vi "Auto Cross.vi"(9 "Defense":T1(ring), 10 "arm":refnum<class "arm.lvclass">, 11 "drive":refnum<class "drive.lvclass">) -> (1 "Stop Wheels":bool, 2 "arm":refnum<class "arm.lvclass">, 3 "drive":refnum<class "drive.lvclass">)   [LabVIEW 2015]
uses:
  drive/drive.lvclass
  arm/arm.lvclass
  <vilib>/Rock Robotics/WPI/RobotDrive/WPI_RobotDriveArcadeDrive_Standard(NoSaturation).vi
  Robot Global Data.vi
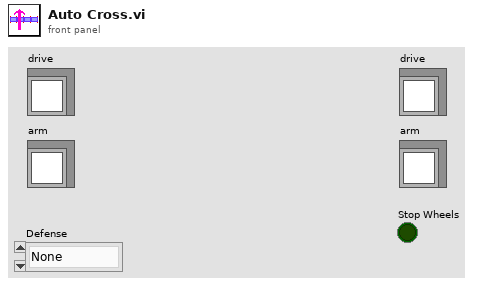
[diagram p1: front panel]
types:
  T1 = enum16{"None", "Low Bar", "Porticullis", "CDF", "Ramparts", "Moat", "Drawbridge", "Sally Port", "Rock Wall", "Rough Terrain"}
  T2 = typedef "WPI_PotentiometerDevRef.ctl" = cluster{"DevStatus":errorcluster, "Analog Channel":T3, "Invert Output":bool}
  T3 = typedef "FPGA_AIChannel.ctl" = enum8{"AI 0", "AI 1", "AI 2", "AI 3", "AI MXP 0", "AI MXP 1", "AI MXP 2", "AI MXP 3", "Invalid"}
  T4 = typedef "WPI_RobotDriveDevRef.ctl" = cluster{"DevStatus":errorcluster, "Motors[]":T5[], "Square Inputs":bool, "Max Output":dbl}
  T5 = typedef "WPI_MotorControlDeviceRef.ctl" = cluster{"DeviceStatus":errorcluster, "Type":T6, "PWM":cluster{"PWM Channel":T7, "DeadBand":T8}, "CAN":cluster{"Device Number":u8, "Control Mode":T9, "Semaphore":T10, "Max Vout":dbl, "TalonSRX Control Mode":T11}, "Invert":bool}
  T6 = typedef "WPI_MotorControlType.ctl" = enum16{"PWM", "CAN", "CANTalonSRX"}
  T7 = typedef "FPGA_DIOPWMChannel.ctl" = enum8{"PWM 0", "PWM 1", "PWM 2", "PWM 3", "PWM 4", "PWM 5", "PWM 6", "PWM 7", "PWM 8", "PWM 9", "PWM MXP 0", "PWM MXP 1", "PWM MXP 2", "PWM MXP 3", "PWM MXP 4", "PWM MXP 5", "PWM MXP 6", "PWM MXP 7", "PWM MXP 8", "PWM MXP 9", "Invalid"}
  T8 = typedef "WPI_PWMDeadband.ctl" = cluster{"Name":string, "maxPositivePwm":i32, "minPositivePwm":i32, "centerPwm":i32, "maxNegativePwm":i32, "minNegativePwm":i32, "angularRange":u16}
  T9 = typedef "WPI_CANJaguar_ControlMode.ctl" = enum8{"Percent VBus", "Current", "Speed", "Position", "Voltage"}
  T10 = typedef "Semaphore RefNum" = refnum<k1>
  T11 = typedef "WPI_CANTalonSRX_APIControlMode.ctl" = enum8{"Percent VBus", "Speed", "Position", "Slave", "Unchanged / Invalid", "Voltage Compensation", "Current", "Motion Profile"}
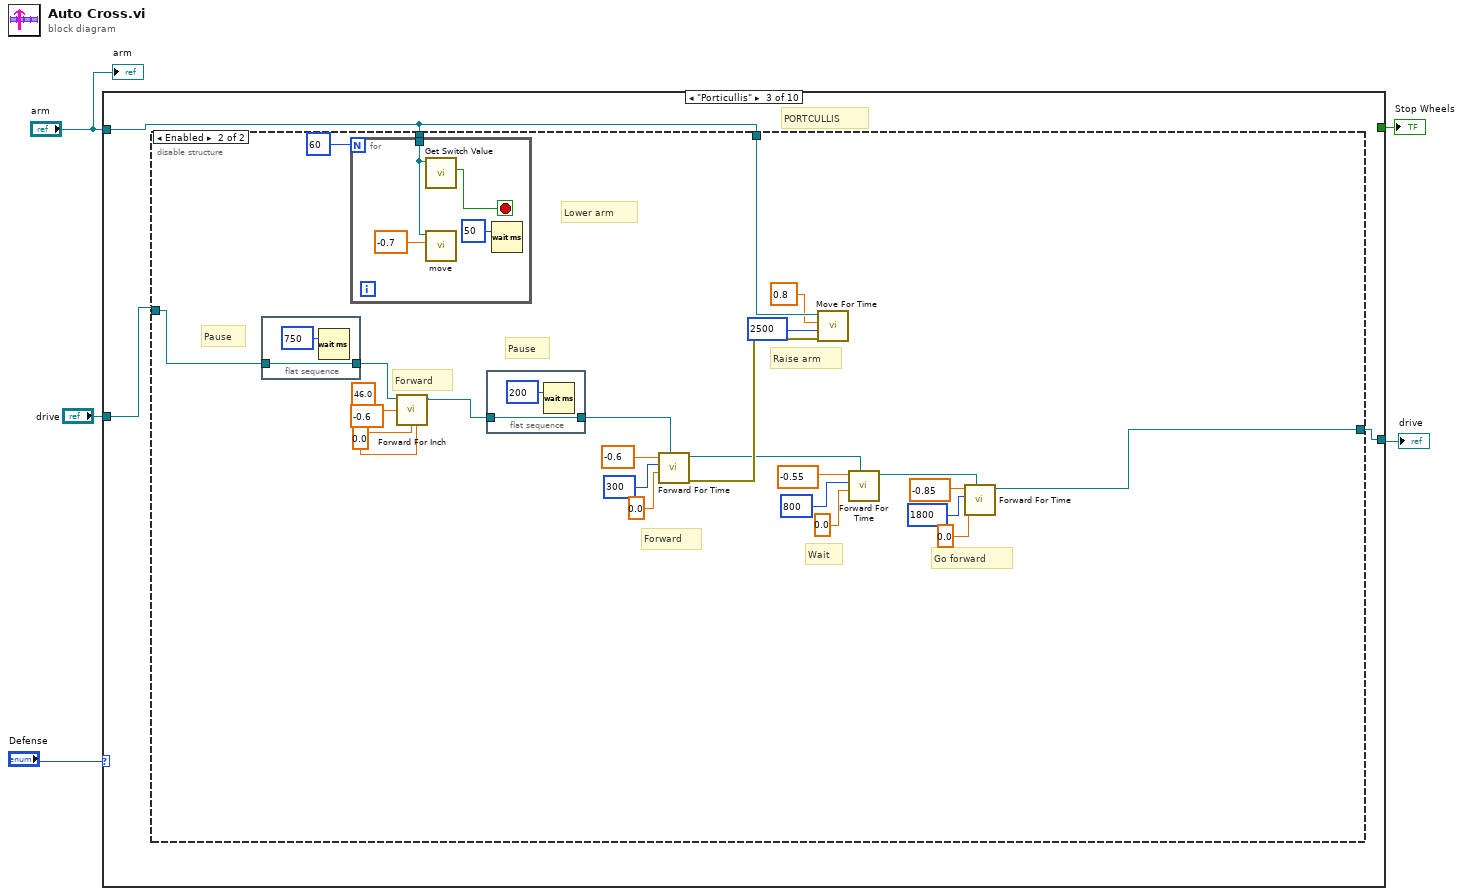
[diagram p0: block diagram]
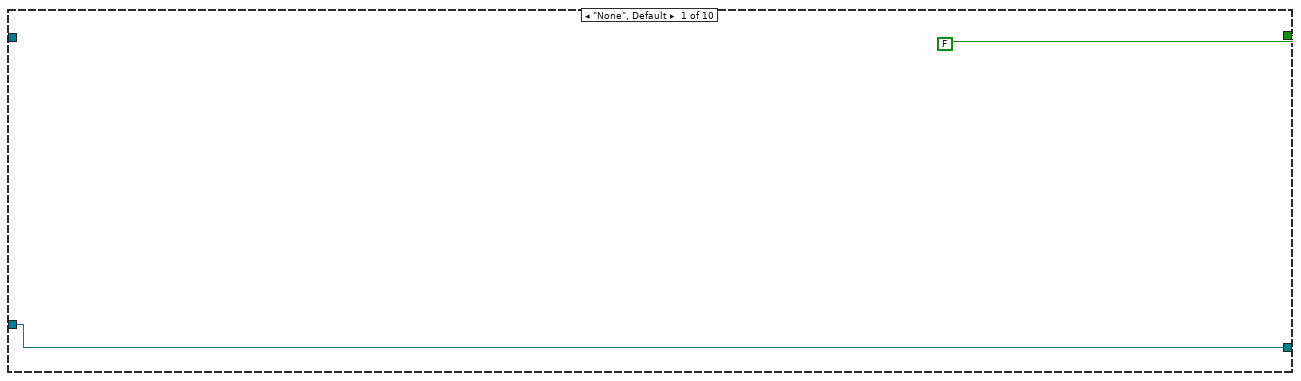
[diagram p2: hidden frame]
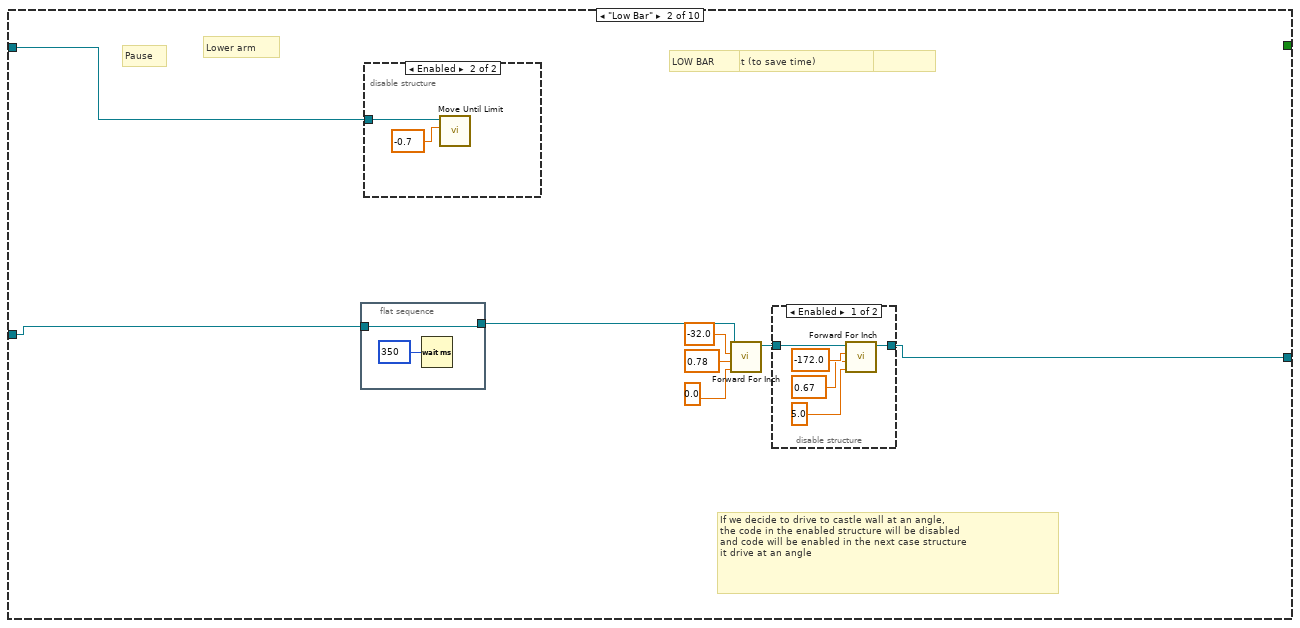
[diagram p3: hidden frame]
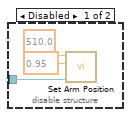
[diagram p5: hidden frame]
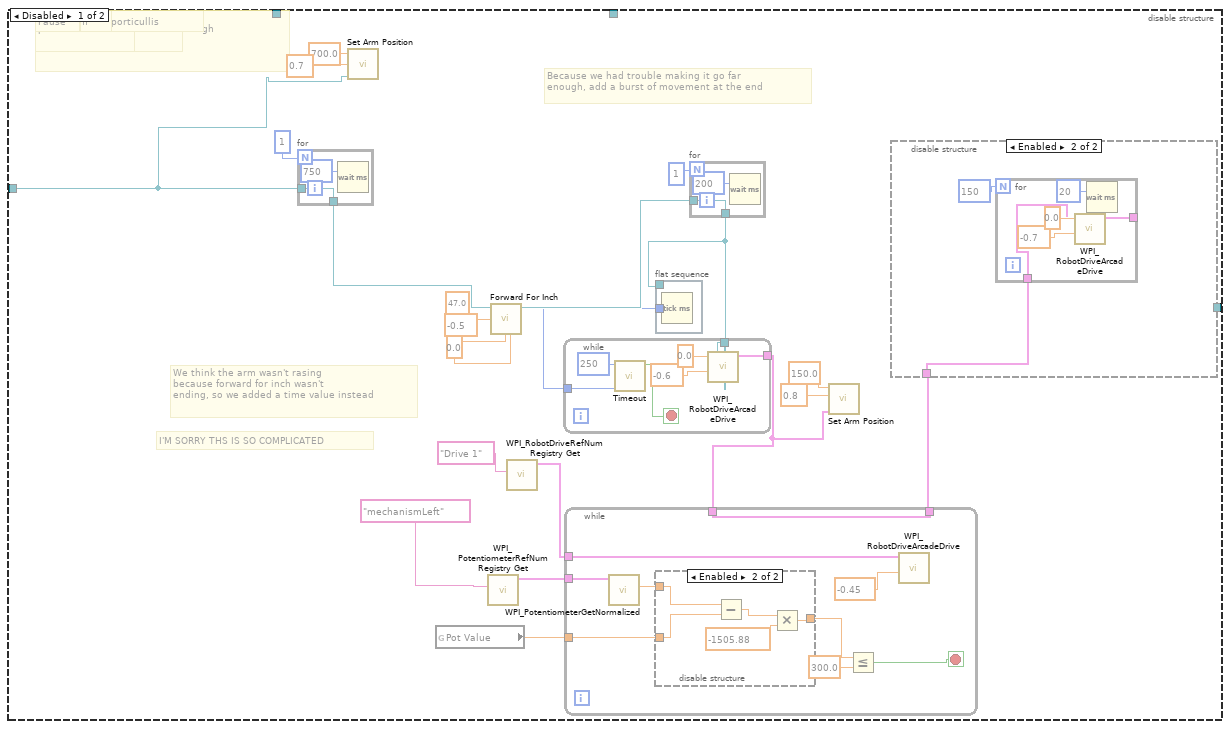
[diagram p6: hidden frame]
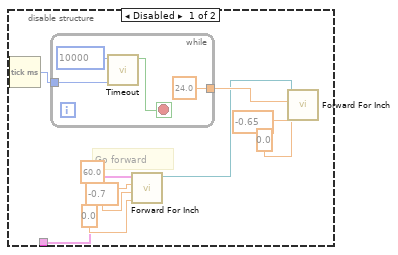
[diagram p7: hidden frame]
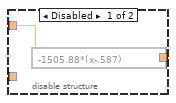
[diagram p8: hidden frame]
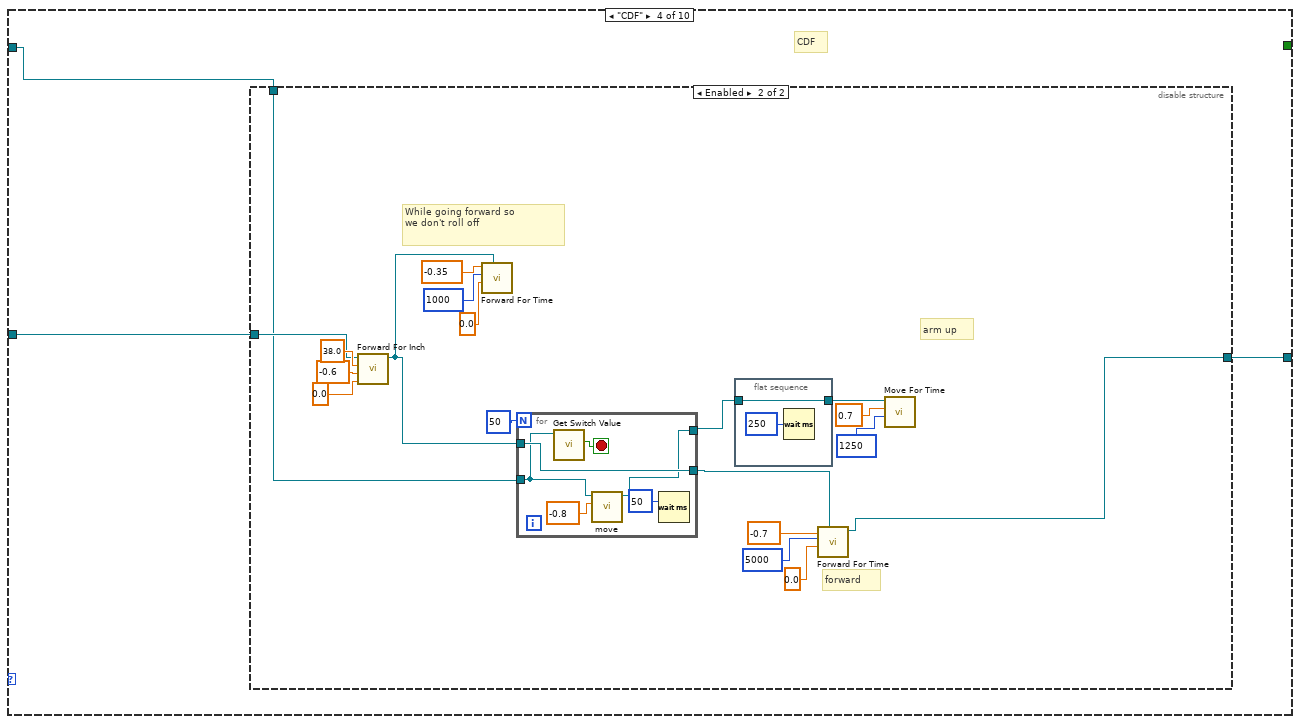
[diagram p9: hidden frame]
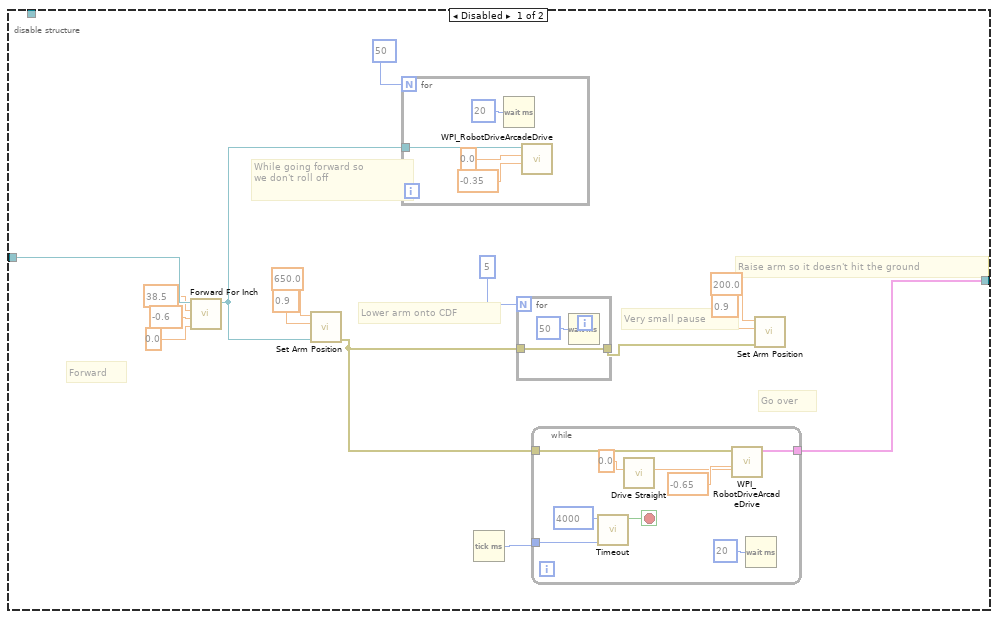
[diagram p10: hidden frame]
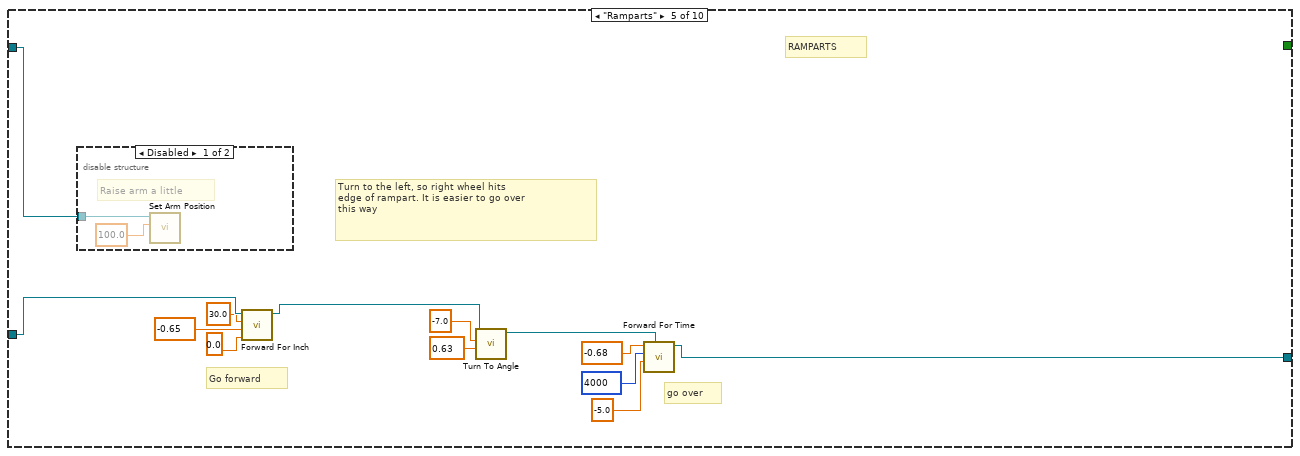
[diagram p11: hidden frame]
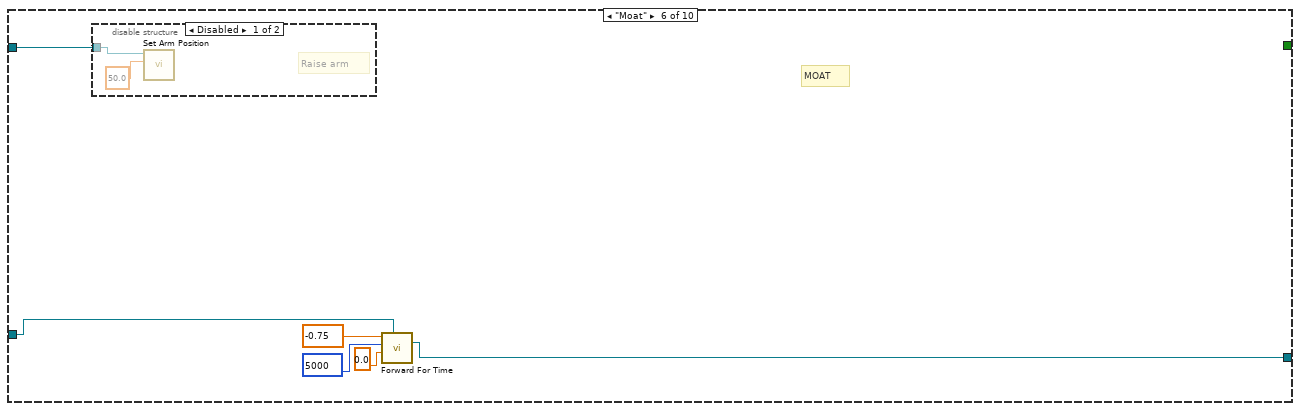
[diagram p13: hidden frame]
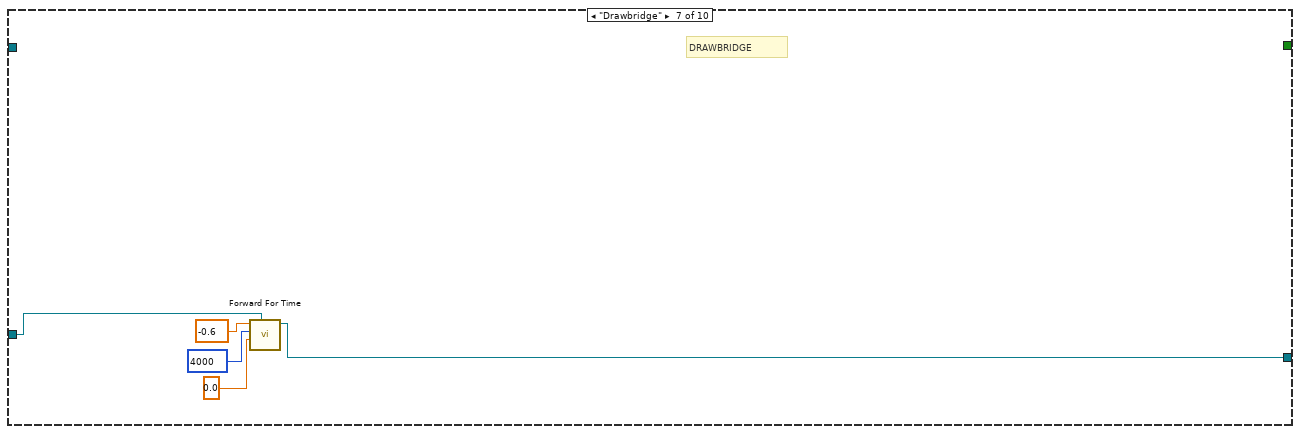
[diagram p15: hidden frame]
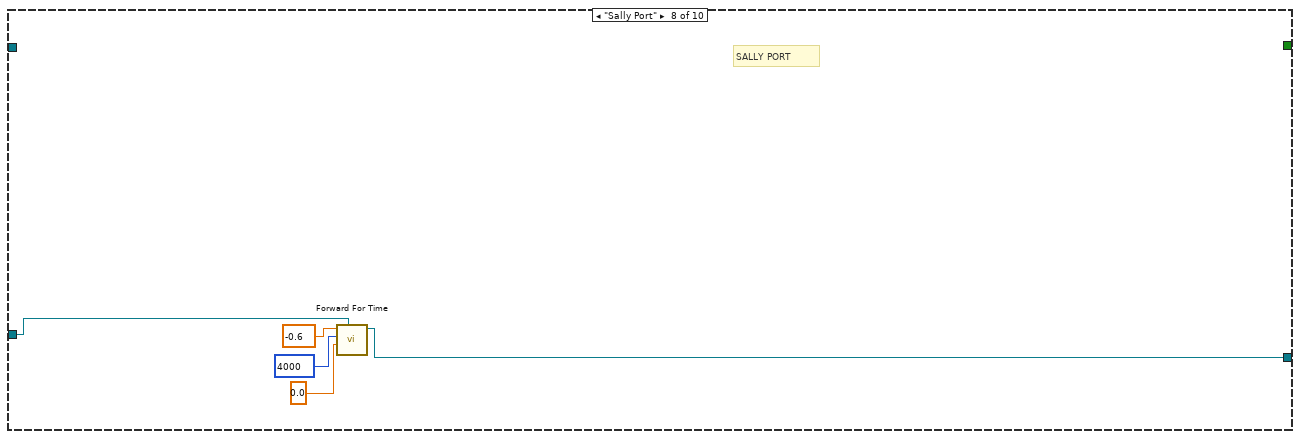
[diagram p16: hidden frame]
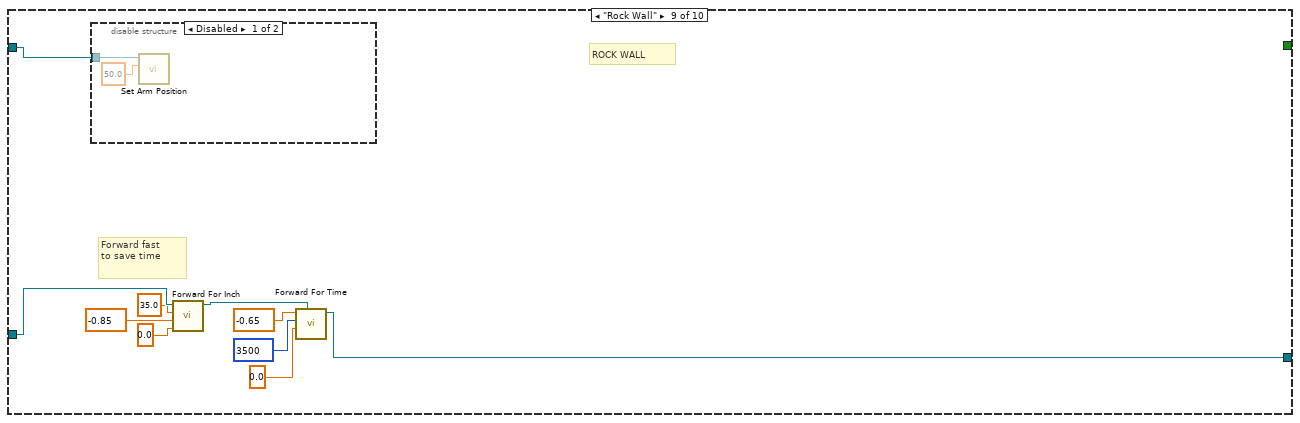
[diagram p17: hidden frame]
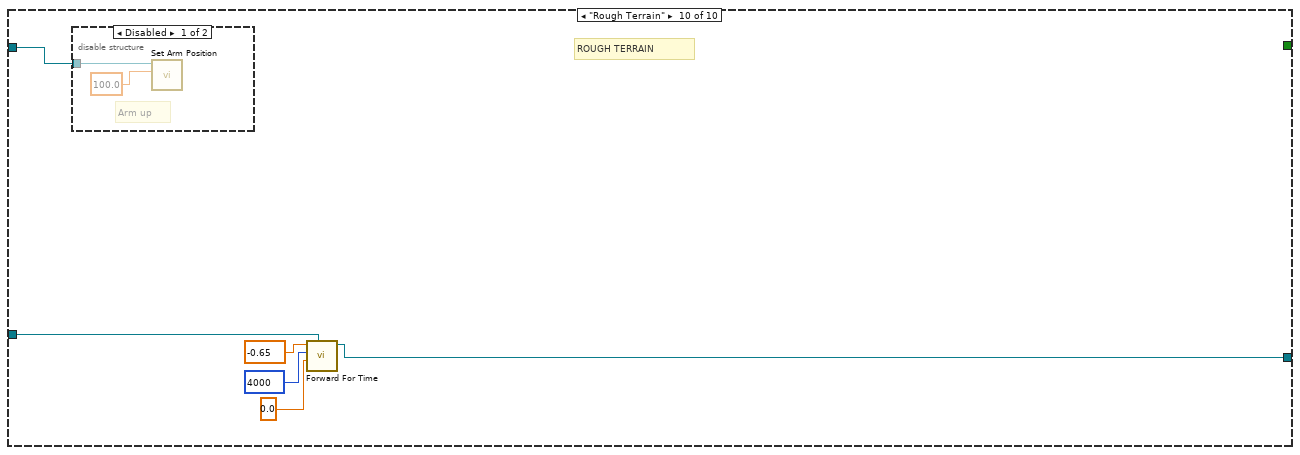
[diagram p19: hidden frame]
diagram:
  n1 = case shown="\"Porticullis\"" "Defense" {
    tunnel: "drive" -> [w6 w10 w31 w136 w204 w214 w218 w223 w236 w240]
    tunnel: [FALSE _ _ _ _ _ _ _ _ _] -> w3
    tunnel: [w6 w11 w29 w134 w194 w210 w217 w222 w227 w239] -> w2
    tunnel: "arm" -> [_ w8 w30 w135 w199 w209 _ _ w232 w244]
    frame "None", Default {
    }
    frame "Low Bar" {
      # "If we decide to drive to castle wall at an angle,\nthe code in the enabled structure will be disabled\nand code will be enabled in the next case structure\nit drive at an angle"
      # "Lower arm"
      # "Go under bar, up to align with low goal"
      # "Go forward fast (to save time)"
      # "Pause"
      # "LOW BAR"
      n2 = flat-sequence {
        tunnel: w10 -> [w16]
        tunnel: [w16] -> w9
        frame #0 {
          n3 = Wait (ms)(milliseconds to wait=u32 350) -> ()  [unwired: 1 out]
        }
      }
      n4 = disable-structure shown="Enabled" {
        disable-tunnel: w8 -> [w26 w28]
        frame Disabled {
          n5 = call "Set Arm Position.vi"("error in (no error)"=w26, "Setpoint"=0.95 ("Speed"), "arm.lvclass"=510.0 ("Setpoint")) -> ()  [unwired: 7 in, 2 out]
        }
        frame Enabled {
          n6 = call "Move Until Limit.vi"("Speed"=-0.7 ("Y axis value"), "arm.lvclass"=w28) -> ()  [unwired: 8 in, 2 out]
        }
      }
      n7 = call "Forward For Inch.vi"("Angle"=0.0 ("Angle robot facing"), "Speed"=0.78, "Distance"=-32.0, "drive.lvclass"=w9) -> ("drive.lvclass"=w12:refnum<class "drive.lvclass">)  [unwired: 6 in, 1 out]
      n8 = disable-structure shown="Enabled" {
        disable-tunnel: [w19 w23] -> w11
        disable-tunnel: w12 -> [w18 w23]
        frame Enabled {
          n9 = call "Forward For Inch.vi"("Angle"=5.0 ("Angle robot facing"), "Speed"=0.67, "Distance"=-172.0, "drive.lvclass"=w18) -> ("drive.lvclass"=w19:refnum<class "drive.lvclass">)  [unwired: 6 in, 1 out]
        }
        frame Disabled {
        }
      }
    }
    frame "Porticullis" {
      # "PORTCULLIS"
      n10 = disable-structure shown="Enabled" {
        disable-tunnel: [_ w102] -> w29
        disable-tunnel: w31 -> [w34 w121]
        disable-tunnel: w30 -> [_ w113]
        disable-tunnel: w30 -> [_ w101]
        frame Disabled {
          # "then pause while arm\nlowering"
          # "Pause"
          # "Because we had trouble making it go far\nenough, add a burst of movement at the end"
          # "We think the arm wasn't rasing\nbecause forward for inch wasn't\nending, so we added a time value instead"
          # "I'M SORRY THS IS SO COMPLICATED"
          # "Go forward slowly, so we \ndon't roll off ramp. When arm is high \nenough, start moving forward"
          # "raise arm, and porticullis"
          # "pause"
          # "Go forward to\nporticullus"
          # "Lower arm"
          n11 = for {
            N: 1 -> [_]
            tunnel: w34 -> [w97]
            tunnel: [w97] -> w45
            n12 = Wait (ms)(milliseconds to wait=u32 750) -> ()  [unwired: 1 out]
          }
          n13 = call "Set Arm Position.vi"("error in (no error)"=w34, "Setpoint"=0.7 ("Speed"), "arm.lvclass"=700.0 ("Setpoint")) -> ()  [unwired: 7 in, 2 out]
          n14 = global read "Robot Global Data.vi" "Pot Value"() -> (w38:dbl)
          n15 = call <vilib>:"WPI_PotentiometerRefNum Registry Get.vi"("refnum name"="mechanismLeft") -> ("PotDevRef"=w39:T2)  [unwired: 9 in, 1 out]
          n16 = call "Forward For Inch.vi"("Angle"=0.0 ("Angle robot facing"), "Speed"=-0.5, "Distance"=47.0, "drive.lvclass"=w45) -> ("drive.lvclass"=w48:refnum<class "drive.lvclass">)  [unwired: 6 in, 1 out]
          n17 = call <vilib>:"WPI_RobotDriveRefNum Registry Get.vi"("refnum name"="Drive 1") -> ("RobotDriveDevRef"=w42:T4)  [unwired: 9 in, 1 out]
          n18 = flat-sequence {
            tunnel: [w53] -> w41
            tunnel: w35 -> [_]
            frame #0 {
              n19 = Tick Count (ms)() -> (millisecond timer value=w53:u32)
            }
          }
          n20 = for {
            N: 1 -> [_]
            tunnel: w48 -> [w99]
            tunnel: [w99] -> w35
            n21 = Wait (ms)(milliseconds to wait=u32 200) -> ()  [unwired: 1 out]
          }
          n22 = while {
            tunnel: w41 -> [w80]
            tunnel: w35 -> [w75]
            tunnel: [w74] -> w36
            stop <- w78 stop-if-true
            n23 = call "Timeout.vi"("Start Time In"=w80, "Time Limit"=u32 250) -> ("Timeout"=w78:bool)  [unwired: 8 in, 1 out]
            n24 = call-poly <vilib>:"WPI_RobotDriveArcadeDrive.vi"("Y axis value"=-0.6, "X axis value"=0.0, "RobotDriveDevRef"=w75) -> ("RobotDriveDevRef"=w74:T4)  [unwired: 6 in, 2 out]
          }
          n25 = while {
            tunnel: w36 -> [w87]
            tunnel: [w87] -> w37
            tunnel: w42 -> [w85]
            tunnel: w39 -> [w84]
            tunnel: w38 -> [w81]
            stop <- w88 stop-if-true
            n26 = call <vilib>:"WPI_PotentiometerGetNormalized.vi"("PotDevRef"=w84) -> ("Normalized Value"=w83:dbl)  [unwired: 8 in, 2 out]
            n27 = disable-structure shown="Enabled" {
              disable-tunnel: w83 -> [w91 w94]
              disable-tunnel: [w90 w92] -> w82
              disable-tunnel: w81 -> [_ w93]
              frame Disabled {
                n28 = expression code="-1505.88*(x-.587)"(w91) -> (w90:dbl)
              }
              frame Enabled {
                n29 = Subtract(x=w94, y=w93) -> (x-y=w96:dbl)
                n30 = Multiply(x=w96, y=-1505.88) -> (x*y=w92:dbl)
              }
            }
            n31 = Less Or Equal?(x=w82, y=300.0) -> (x <= y?=w88:bool)
            n32 = call-poly <vilib>:"WPI_RobotDriveArcadeDrive.vi"("Y axis value"=-0.45, "RobotDriveDevRef"=w85) -> ()  [unwired: 7 in, 3 out]
          }
          n33 = call "Set Arm Position.vi"("error in (no error)"=w36, "Setpoint"=0.8 ("Speed"), "arm.lvclass"=150.0 ("Setpoint")) -> ()  [unwired: 7 in, 2 out]
          n34 = disable-structure shown="Enabled" {
            disable-tunnel: w37 -> [w54 w67]
            frame Disabled {
              # "Go forward"
              n35 = Tick Count (ms)() -> (millisecond timer value=w59:u32)
              n36 = while {
                tunnel: w59 -> [w66]
                tunnel: [24.0 ("Distance")] -> w56
                stop <- w64 stop-if-true
                n37 = call "Timeout.vi"("Start Time In"=w66, "Time Limit"=u32 10000) -> ("Timeout"=w64:bool)  [unwired: 8 in, 1 out]
              }
              n38 = call "Forward For Inch.vi"("Angle"=0.0 ("Angle robot facing"), "Speed"=-0.7, "Distance"=60.0, "drive.lvclass"=w54) -> ("drive.lvclass"=w55:refnum<class "drive.lvclass">)  [unwired: 6 in, 1 out]
              n39 = call "Forward For Inch.vi"("Angle"=0.0 ("Angle robot facing"), "Speed"=-0.65, "Distance"=w56, "drive.lvclass"=w55) -> ()  [unwired: 6 in, 2 out]
            }
            frame Enabled {
              n40 = for {
                N: 150 -> [_]
                tunnel: w67 -> [w71]
                tunnel: [w69] -> _
                n41 = call-poly <vilib>:"WPI_RobotDriveArcadeDrive.vi"("Y axis value"=-0.7, "X axis value"=0.0, "RobotDriveDevRef"=w71) -> ("RobotDriveDevRef"=w69:T4)  [unwired: 6 in, 2 out]
                n42 = Wait (ms)(milliseconds to wait=u32 20) -> ()  [unwired: 1 out]
              }
            }
          }
        }
        frame Enabled {
          # "Go forward"
          # "Wait"
          # "Raise arm"
          # "Forward"
          # "Pause"
          # "Forward"
          # "Lower arm"
          # "Pause"
          n43 = flat-sequence {
            tunnel: w121 -> [w128]
            tunnel: [w128] -> w120
            frame #0 {
              n44 = Wait (ms)(milliseconds to wait=u32 750) -> ()  [unwired: 1 out]
            }
          }
          n45 = for {
            N: 60 -> [_]
            tunnel: w101 -> [w130]
            stop <- w132 stop-if-true
            n46 = call "Get Switch Value.vi"("arm.lvclass"=w130) -> ("Switch Pressed"=w132:bool)  [unwired: 9 in, 1 out]
            n47 = call "move.vi"("Speed"=-0.7 ("Y axis value"), "arm.lvclass"=w130) -> ()  [unwired: 9 in, 1 out]
            n48 = Wait (ms)(milliseconds to wait=u32 50) -> ()  [unwired: 1 out]
          }
          n49 = call "Forward For Inch.vi"("Angle"=0.0 ("Angle robot facing"), "Speed"=-0.6, "Distance"=46.0, "drive.lvclass"=w120) -> ("drive.lvclass"=w119:refnum<class "drive.lvclass">)  [unwired: 6 in, 1 out]
          n50 = flat-sequence {
            tunnel: w119 -> [w126]
            tunnel: [w126] -> w118
            frame #0 {
              n51 = Wait (ms)(milliseconds to wait=u32 200) -> ()  [unwired: 1 out]
            }
          }
          n52 = call "Forward For Time.vi"("drive.lvclass"=w118, "Angle"=0.0, "Time (ms)"=u32 300 ("milliseconds to wait"), "Speed"=-0.6 ("Y axis value")) -> ("error out"=w114:errorcluster, "drive.lvclass"=w110:refnum<class "drive.lvclass">)  [unwired: 6 in]
          n53 = call "Move For Time.vi"("error in (no error)"=w114, "Time (ms)"=u32 2500 ("milliseconds to wait"), "Speed"=0.8 ("Y axis value"), "arm.lvclass"=w113) -> ()  [unwired: 6 in, 2 out]
          n54 = call "Forward For Time.vi"("drive.lvclass"=w110, "Angle"=0.0, "Time (ms)"=u32 800, "Speed"=-0.55 ("Y axis value")) -> ("drive.lvclass"=w106:refnum<class "drive.lvclass">)  [unwired: 6 in, 1 out]
          n55 = call "Forward For Time.vi"("drive.lvclass"=w106, "Angle"=0.0, "Time (ms)"=u32 1800 ("milliseconds to wait"), "Speed"=-0.85 ("Y axis value")) -> ("drive.lvclass"=w102:refnum<class "drive.lvclass">)  [unwired: 6 in, 1 out]
        }
      }
    }
    frame "CDF" {
      # "CDF"
      n56 = disable-structure shown="Enabled" {
        disable-tunnel: w136 -> [w151 w182]
        disable-tunnel: [w137 w170] -> w134
        disable-tunnel: w135 -> [_ w172]
        frame Disabled {
          # "Raise arm so it doesn't hit the ground"
          # "Go over"
          # "Very small pause"
          # "While going forward so\nwe don't roll off"
          # "Lower arm onto CDF"
          # "Forward"
          n57 = call "Forward For Inch.vi"("Angle"=0.0 ("Angle robot facing"), "Speed"=-0.6, "Distance"=38.5, "drive.lvclass"=w151) -> ("drive.lvclass"=w142:refnum<class "drive.lvclass">)  [unwired: 6 in, 1 out]
          n58 = call "Set Arm Position.vi"("error in (no error)"=w142, "Setpoint"=0.9 ("Speed"), "arm.lvclass"=650.0 ("Setpoint")) -> ("error out (no error)"=w141:errorcluster)  [unwired: 7 in, 1 out]
          n59 = for {
            N: 50 -> [_]
            tunnel: w142 -> [w154]
            n60 = Wait (ms)(milliseconds to wait=u32 20) -> ()  [unwired: 1 out]
            n61 = call-poly <vilib>:"WPI_RobotDriveArcadeDrive.vi"("Y axis value"=-0.35, "X axis value"=0.0 ("Y axis value"), "RobotDriveDevRef"=w154) -> ()  [unwired: 6 in, 3 out]
          }
          n62 = Tick Count (ms)() -> (millisecond timer value=w138:u32)
          n63 = for {
            N: 5 -> [_]
            tunnel: [w152] -> w143
            tunnel: w141 -> [w152]
            n64 = Wait (ms)(milliseconds to wait=u32 50) -> ()  [unwired: 1 out]
          }
          n65 = while {
            tunnel: w141 -> [w165]
            tunnel: [w164] -> w137
            tunnel: w138 -> [w161]
            stop <- w160 stop-if-true
            n66 = call "Timeout.vi"("Start Time In"=w161, "Time Limit"=u32 4000) -> ("Timeout"=w160:bool)  [unwired: 8 in, 1 out]
            n67 = call "Drive Straight.vi"("Angle robot facing"=0.0) -> ("Arcade drive x"=w158:dbl)  [unwired: 9 in, 1 out]
            n68 = call-poly <vilib>:"WPI_RobotDriveArcadeDrive.vi"("Y axis value"=-0.65, "X axis value"=w158, "RobotDriveDevRef"=w165) -> ("RobotDriveDevRef"=w164:T4)  [unwired: 6 in, 2 out]
            n69 = Wait (ms)(milliseconds to wait=u32 20) -> ()  [unwired: 1 out]
          }
          n70 = call "Set Arm Position.vi"("error in (no error)"=w143, "Setpoint"=0.9 ("Speed"), "arm.lvclass"=200.0 ("Setpoint")) -> ()  [unwired: 7 in, 2 out]
        }
        frame Enabled {
          # "forward"
          # "arm up"
          # "While going forward so\nwe don't roll off"
          n71 = call "Forward For Inch.vi"("Angle"=0.0 ("Angle robot facing"), "Speed"=-0.6, "Distance"=38.0, "drive.lvclass"=w182) -> ("drive.lvclass"=w180:refnum<class "drive.lvclass">)  [unwired: 6 in, 1 out]
          n72 = call "Forward For Time.vi"("drive.lvclass"=w180, "Angle"=0.0, "Time (ms)"=u32 1000 ("milliseconds to wait"), "Speed"=-0.35 ("Y axis value")) -> ()  [unwired: 6 in, 2 out]
          n73 = for {
            N: 50 -> [_]
            tunnel: w172 -> [w189]
            tunnel: w180 -> [w192]
            tunnel: [w191] -> w176
            tunnel: [w192] -> w171
            stop <- w190 stop-if-true
            n74 = call "Get Switch Value.vi"("arm.lvclass"=w189) -> ("Switch Pressed"=w190:bool)  [unwired: 9 in, 1 out]
            n75 = call "move.vi"("Speed"=-0.8 ("Y axis value"), "arm.lvclass"=w189) -> ("arm.lvclass"=w191:refnum<class "arm.lvclass">)  [unwired: 9 in]
            n76 = Wait (ms)(milliseconds to wait=u32 50) -> ()  [unwired: 1 out]
          }
          n77 = flat-sequence {
            tunnel: w176 -> [w186]
            tunnel: [w186] -> w175
            frame #0 {
              n78 = Wait (ms)(milliseconds to wait=u32 250) -> ()  [unwired: 1 out]
            }
          }
          n79 = call "Forward For Time.vi"("drive.lvclass"=w171, "Angle"=0.0, "Time (ms)"=u32 5000 ("Time Limit"), "Speed"=-0.7 ("Y axis value")) -> ("drive.lvclass"=w170:refnum<class "drive.lvclass">)  [unwired: 6 in, 1 out]
          n80 = call "Move For Time.vi"("Time (ms)"=u32 1250 ("milliseconds to wait"), "Speed"=0.7 ("Y axis value"), "arm.lvclass"=w175) -> ()  [unwired: 7 in, 2 out]
        }
      }
    }
    frame "Ramparts" {
      # "go over"
      # "Turn to the left, so right wheel hits\nedge of rampart. It is easier to go over\nthis way"
      # "Go forward"
      # "RAMPARTS"
      n81 = disable-structure shown="Disabled" {
        disable-tunnel: w199 -> [w208 _]
        frame Disabled {
          # "Raise arm a little"
          n82 = call "Set Arm Position.vi"("Setpoint"=100.0, "arm.lvclass"=w208) -> ()  [unwired: 8 in, 2 out]
        }
        frame Enabled {
        }
      }
      n83 = call "Forward For Inch.vi"("Angle"=0.0 ("Angle robot facing"), "Speed"=-0.65, "Distance"=30.0, "drive.lvclass"=w204) -> ("drive.lvclass"=w200:refnum<class "drive.lvclass">)  [unwired: 6 in, 1 out]
      n84 = call "Turn To Angle.vi"("Speed/Direction"=0.63, "Angle"=-7.0, "drive.lvclass"=w200) -> ("drive.lvclass"=w195:refnum<class "drive.lvclass">)  [unwired: 7 in, 1 out]
      n85 = call "Forward For Time.vi"("drive.lvclass"=w195, "Angle"=-5.0 ("Angle robot facing"), "Time (ms)"=u32 4000 ("Time Limit"), "Speed"=-0.68 ("Y axis value")) -> ("drive.lvclass"=w194:refnum<class "drive.lvclass">)  [unwired: 6 in, 1 out]
    }
    frame "Moat" {
      # "MOAT"
      n86 = disable-structure shown="Disabled" {
        disable-tunnel: w209 -> [w215 _]
        frame Disabled {
          # "Raise arm"
          n87 = call "Set Arm Position.vi"("Setpoint"=50.0, "arm.lvclass"=w215) -> ()  [unwired: 8 in, 2 out]
        }
        frame Enabled {
        }
      }
      n88 = call "Forward For Time.vi"("drive.lvclass"=w214, "Angle"=0.0, "Time (ms)"=u32 5000 ("Time Limit"), "Speed"=-0.75 ("Y axis value")) -> ("drive.lvclass"=w210:refnum<class "drive.lvclass">)  [unwired: 6 in, 1 out]
    }
    frame "Drawbridge" {
      # "DRAWBRIDGE"
      n89 = call "Forward For Time.vi"("drive.lvclass"=w218, "Angle"=0.0 ("Angle robot facing"), "Time (ms)"=u32 4000 ("Time Limit"), "Speed"=-0.6 ("Y axis value")) -> ("drive.lvclass"=w217:refnum<class "drive.lvclass">)  [unwired: 6 in, 1 out]
    }
    frame "Sally Port" {
      # "SALLY PORT"
      n90 = call "Forward For Time.vi"("drive.lvclass"=w223, "Angle"=0.0 ("Angle robot facing"), "Time (ms)"=u32 4000 ("Time Limit"), "Speed"=-0.6 ("Y axis value")) -> ("drive.lvclass"=w222:refnum<class "drive.lvclass">)  [unwired: 6 in, 1 out]
    }
    frame "Rock Wall" {
      # "ROCK WALL"
      # "Forward fast\nto save time"
      n91 = disable-structure shown="Disabled" {
        disable-tunnel: w232 -> [w238 _]
        frame Disabled {
          n92 = call "Set Arm Position.vi"("Setpoint"=50.0, "arm.lvclass"=w238) -> ()  [unwired: 8 in, 2 out]
        }
        frame Enabled {
        }
      }
      n93 = call "Forward For Inch.vi"("Angle"=0.0 ("Angle robot facing"), "Speed"=-0.85, "Distance"=35.0, "drive.lvclass"=w236) -> ("drive.lvclass"=w228:refnum<class "drive.lvclass">)  [unwired: 6 in, 1 out]
      n94 = call "Forward For Time.vi"("drive.lvclass"=w228, "Angle"=0.0 ("Angle robot facing"), "Time (ms)"=u32 3500 ("Time Limit"), "Speed"=-0.65 ("Y axis value")) -> ("drive.lvclass"=w227:refnum<class "drive.lvclass">)  [unwired: 6 in, 1 out]
    }
    frame "Rough Terrain" {
      # "ROUGH TERRAIN"
      n95 = disable-structure shown="Disabled" {
        disable-tunnel: w244 -> [w246 _]
        frame Disabled {
          # "Arm up"
          n96 = call "Set Arm Position.vi"("Setpoint"=100.0, "arm.lvclass"=w246) -> ()  [unwired: 8 in, 2 out]
        }
        frame Enabled {
        }
      }
      n97 = call "Forward For Time.vi"("drive.lvclass"=w240, "Angle"=0.0 ("Angle robot facing"), "Time (ms)"=u32 4000 ("Time Limit"), "Speed"=-0.65 ("Y axis value")) -> ("drive.lvclass"=w239:refnum<class "drive.lvclass">)  [unwired: 6 in, 1 out]
    }
  }
  "drive" <- w2
  "Stop Wheels" <- w3
  "arm" <- "arm"
